vi "Vision Processing.vi"(4 "error in (no error)":errorcluster, 5 "Camera Type":enum16{"206", "1011"}(ring), 6 "Camera Name":string="Camera") -> (0 "Target Info":T1(array[cluster]), 2 "Processed Image":T3(plugin-control))   [LabVIEW 2013]
uses:
  Robot Global Data.vi
  <vilib>/vision/NI_Vision_Development_Module.lvlib
panel:
  in  "View":bool
  in  "Area Size Limit":i32=444
  in  "Particle Count Limit":i32=8
  in  "Score Limits":T2={"Rect Coverage"=76.0, "Aspect Ratio"=70.0, "X Edge Strength"=40.0, "Y Edge Strength"=60.0}
  in  "Processing":enum32{"Color", "Intensity", "Intensity Open"}(tab)
  in  "Luminance":i32=255
  in  "Saturation":i32=255
  in  "Hue":i32(knob)=65 scale=0.0..255.0
  in  "Margins":cluster{"Hue":i32, "Sat":i32, "Lum":i32}={"Hue"=20, "Sat"=27, "Lum"=30} {"Sat" scale=0.0..40.0; "Lum" scale=0.0..40.0; "Hue" scale=0.0..40.0}
  in  "Range":cluster{"Lower value":sgl, "Upper value":sgl}={"Lower value"=150.0, "Upper value"=255.0} {"Lower value" scale=0.0..255.0; "Upper value" scale=0.0..255.0}
  in  "Range":cluster{"Lower value":sgl, "Upper value":sgl}={"Lower value"=150.0, "Upper value"=255.0} {"Lower value" scale=0.0..255.0; "Upper value" scale=0.0..255.0}
  in  "View":bool
  out "Original Image":T3(plugin-control)
  # "Instructions:\nProcessing the reflective tape that is illuminated by a ring light can be based\non color or light intensity.\nParticles within the image are scored by rectangle coverage, aspect ratio, and\nfor being hollow with a bold edge. A particle is considered a target if all scores\nare above the score limits. Particles can be annotated -- surrounded by\na rectangle and scores drawn to the left .\nTo control the number of particles being scored, use the count limit and the size\nlimit."
  # "To debug, Enable using the View button.\nFor color processing, you can click in the image to select the color for processing."
  # "Enable by clicking the View button.\nGreen scores are above the limit, orange are below. Inner/outer rect\nindicates all passed."
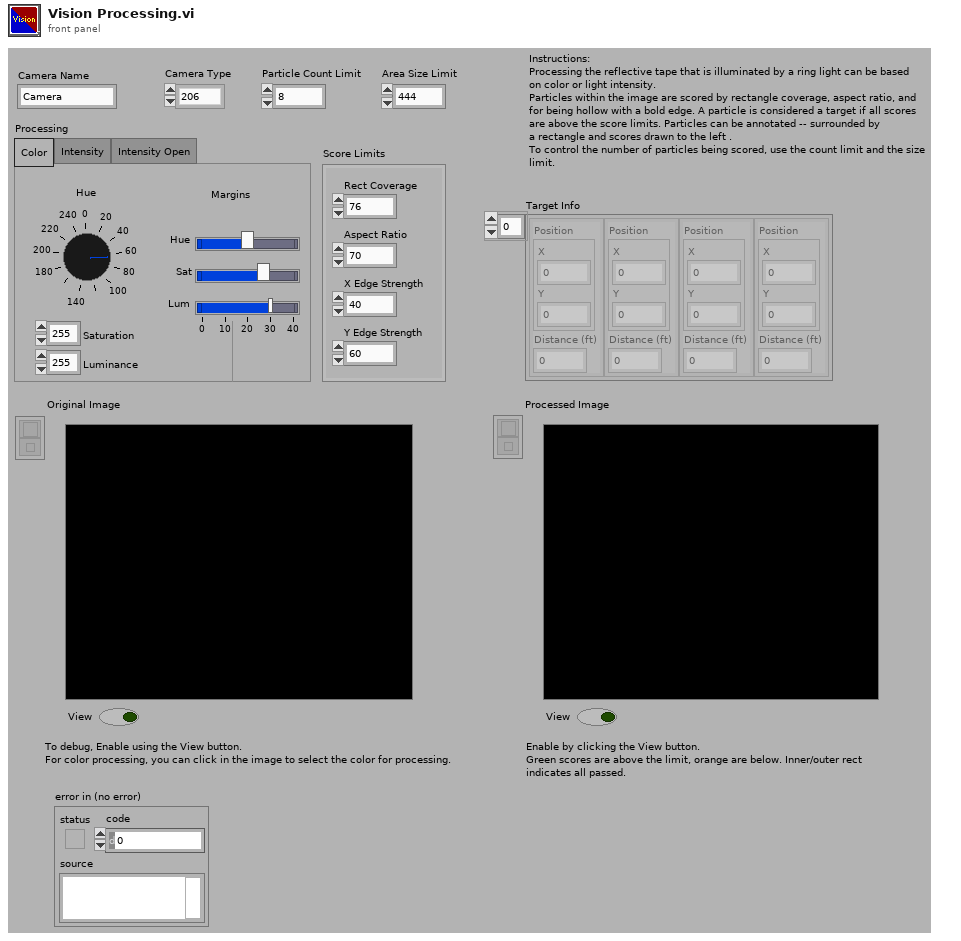
[diagram p1: front panel]
types:
  T1 = cluster{"Position":cluster{"X":dbl, "Y":dbl}, "Distance (ft)":dbl}[]
  T2 = cluster{"Rect Coverage":dbl, "Aspect Ratio":dbl, "X Edge Strength":dbl, "Y Edge Strength":dbl}
  T3 = typedef "IMAQ Image.ctl" = refnum<image>
  T4 = typedef "Image Type" = u32
  T5 = typedef "WPI_CameraDevRef.ctl" = cluster{"Camera Address":string, "CameraStatus":errorcluster, "Acquire Image Notifier":refnum<notifier>}
  T6 = enum32{"AutoM", "Close", "Dilate", "Erode", "Gradient", "Gradient out", "Gradient in", "Hit miss", "Open", "PClose", "POpen", "Thick", "Thin"}
  T7 = typedef "WPI_CameraImageSize.ctl" = enum16{"640x480", "320x240", "160x120"}
  T8 = cluster{cluster{"Left":dbl, "Top":dbl, "Right":dbl, "Bottom":dbl}, dbl[]}[]
  T9 = cluster{"Left":dbl, "Top":dbl, "Right":dbl, "Bottom":dbl}
  T10 = cluster{"Target Center (-1 to 1)":cluster{"X":dbl, "Y":dbl}, "Distance (ft)":dbl}
  T11 = cluster{"Target Center (-1 to 1)":cluster{"X":dbl, "Y":dbl}, "Distance (ft)":dbl}[]
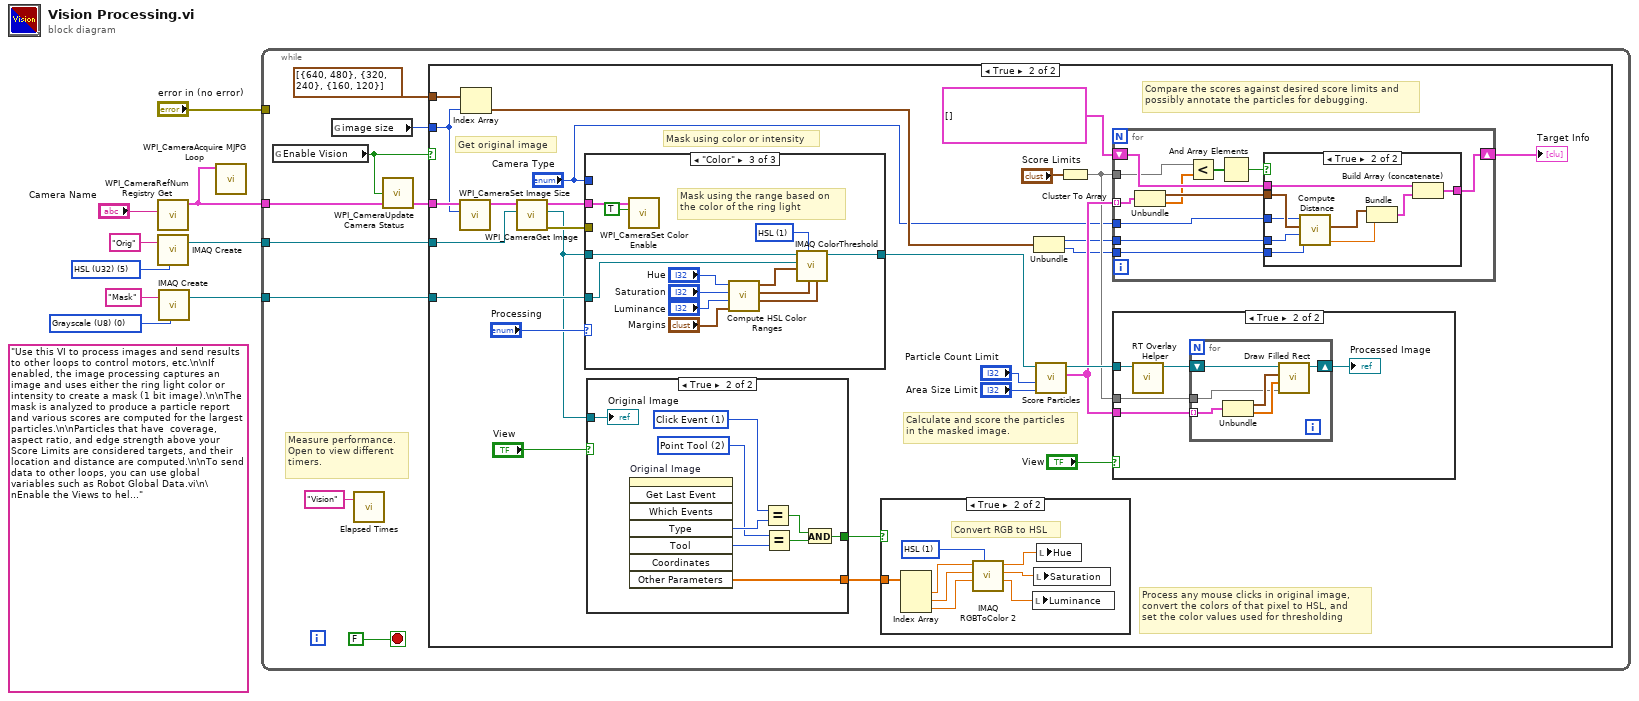
[diagram p0: block diagram]
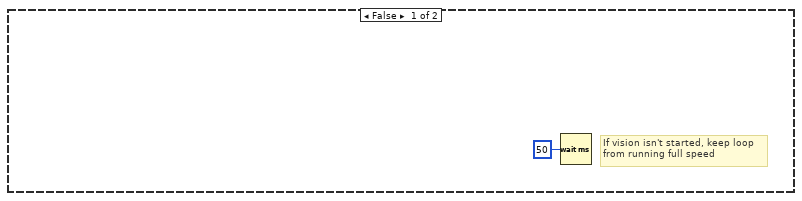
[diagram p2: hidden frame]
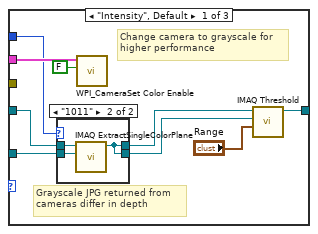
[diagram p4: hidden frame]
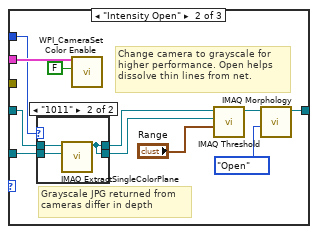
[diagram p6: hidden frame]
diagram:
  w3 = T4 0 items=["Grayscale (U8)", "Grayscale (I16)", "Grayscale (SGL)", "Complex (CSG)", "RGB (U32)", "HSL (U32)", "RGB (U64)", "Grayscale (U16)"] ("Image Type")
  (unwired) "Use this VI to process images and send results to other loops to control motors, etc.\n\nIf enabled, the image processing captures an image and uses either the ring light color or intensity to create a mask (1 bit image).\n\nThe mask is analyzed to produce a particle report and various scores are computed for the largest particles.\n\nParticles that have  coverage, aspect ratio, and edge strength above your Score Limits are considered targets, and their location and distance are computed.\n\nTo send data to other loops, you can use global variables such as Robot Global Data.vi\n\nEnable the Views to help debug color settings. Disable the View to speed up processing."
  w8 = T4 5 items=["Grayscale (U8)", "Grayscale (I16)", "Grayscale (SGL)", "Complex (CSG)", "RGB (U32)", "HSL (U32)", "RGB (U64)", "Grayscale (U16)"] ("Image Type")
  n1 = call <vilib>:"WPI_CameraRefNum Registry Get.vi"("refnum name"="Camera Name") -> ("CameraDevRef"=w5:T5)  [unwired: 9 in, 1 out]
  n2 = call "IMAQ Create"("Image Name"="Orig", "Image Type"=w8) -> ("New Image"=w7:T3)  [unwired: 2 in, 2 out]
  n3 = call "IMAQ Create"("Image Name"="Mask", "Image Type"=w3) -> ("New Image"=w1:T3)  [unwired: 2 in, 2 out]
  n4 = call <vilib>:"WPI_CameraAcquire MJPG Loop.vi"("CameraDevRef"=w5) -> ()  [unwired: 11 in]
  n5 = while {
    tunnel: w7 -> [w17]
    tunnel: w5 -> [w16]
    tunnel: "error in (no error)" -> [_]
    tunnel: w1 -> [w11]
    stop <- FALSE stop-if-true
    # "Measure performance.\nOpen to view different\ntimers."
    n6 = global read "Robot Global Data.vi" "Enable Vision"() -> (w14:bool)
    n7 = global read "Robot Global Data.vi" "image size"() -> (w12:T7)
    n8 = call "Elapsed Times.vi"("Call Name"="Vision") -> ()  [unwired: 2 in, 1 out]
    n9 = call <vilib>:"WPI_CameraUpdate Camera Status.vi"("CameraDevRef In"=w16, "Enable Vision"=w14) -> ("CameraDevRef Out"=w15:T5)  [unwired: 3 in]
    n10 = case shown="True" w14 {
      tunnel: w17 -> [_ w37]
      tunnel: w15 -> [_ w33]
      tunnel: w12 -> [_ w28]
      tunnel: w11 -> [_ w23]
      tunnel: cluster{i32, i32}[] [{640, 480}, {320, 240}, {160, 120}] -> [_ w27]
      frame False {
        # "If vision isn't started, keep loop\nfrom running full speed"
        n11 = Wait (ms)(milliseconds to wait=u32 50) -> ()  [unwired: 1 out]
      }
      frame True {
        # "Compare the scores against desired score limits and\npossibly annotate the particles for debugging."
        # "Process any mouse clicks in original image,\nconvert the colors of that pixel to HSL, and\nset the color values used for thresholding"
        # "Calculate and score the particles\nin the masked image."
        # "Mask using color or intensity"
        # "Get original image"
        n12 = call <vilib>:"WPI_CameraSet Image Size.vi"("Image Size"=w28, "CameraDevRef"=w33) -> ("CameraDevRef Out"=w34:T5)  [unwired: 8 in, 1 out]
        n13 = Index Array(array=w27, index=w28) -> (element=w24:cluster{i32, i32})
        n14 = call <vilib>:"WPI_CameraGet Image.vi"("Image"=w37, "CameraDevRef"=w34) -> ("error out"=w35:errorcluster, "Image Out"=w22:T3, "CameraDevRef Out"=w36:T5)  [unwired: 7 in]
        n15 = case shown="\"Color\"" "Processing" {
          tunnel: w22 -> [w59 w71 w97]
          tunnel: [w62 w76 w96] -> w31
          tunnel: w36 -> [w60 w74 w87]
          tunnel: w35 -> [_ _ _]
          tunnel: w23 -> [w58 w72 w85]
          tunnel: "Camera Type" -> [w57 w73 _]
          frame "Intensity", Default {
            # "Grayscale JPG returned from\ncameras differ in depth"
            # "Change camera to grayscale for\nhigher performance"
            n16 = case shown="\"1011\"" w57 {
              tunnel: w59 -> [w65 w68]
              tunnel: w58 -> [w64 w67]
              tunnel: [w65 w66] -> w56
              tunnel: [w64 w66] -> w55
              frame "206", Default {
              }
              frame "1011" {
                n17 = call "IMAQ ExtractSingleColorPlane"("Image Dst"=w67, "Image Src"=w68) -> ("Image Dst Out"=w66:T3)  [unwired: 8 in, 1 out]
              }
            }
            n18 = call <vilib>:"WPI_CameraSet Color Enable.vi"("Color Enabled"=FALSE, "CameraDevRef"=w60) -> ()  [unwired: 8 in, 2 out]
            n19 = call "IMAQ Threshold"("Range"="Range", "Image Dst"=w55, "Image Src"=w56) -> ("Image Dst Out"=w62:T3)  [unwired: 3 in, 5 out]
          }
          frame "Intensity Open" {
            # "Grayscale JPG returned from\ncameras differ in depth"
            # "Change camera to grayscale for\nhigher performance. Open helps\ndissolve thin lines from net."
            n20 = case shown="\"1011\"" w73 {
              tunnel: w71 -> [w81 w84]
              tunnel: w72 -> [w80 w83]
              tunnel: [w81 w82] -> w70
              tunnel: [w80 w82] -> w69
              frame "206", Default {
              }
              frame "1011" {
                n21 = call "IMAQ ExtractSingleColorPlane"("Image Dst"=w83, "Image Src"=w84) -> ("Image Dst Out"=w82:T3)  [unwired: 8 in, 1 out]
              }
            }
            n22 = call <vilib>:"WPI_CameraSet Color Enable.vi"("Color Enabled"=FALSE, "CameraDevRef"=w74) -> ()  [unwired: 8 in, 2 out]
            n23 = call "IMAQ Threshold"("Range"="Range", "Image Dst"=w69, "Image Src"=w70) -> ("Image Dst Out"=w77:T3)  [unwired: 3 in, 5 out]
            n24 = call "IMAQ Morphology"("Operation"=T6."Open", "Image Src"=w77) -> ("Image Dst Out"=w76:T3)  [unwired: 8 in, 1 out]
          }
          frame "Color" {
            w95 = u16 1 items=["RGB", "HSL", "HSV", "HSI"] ("Color Mode")
            # "Mask using the range based on\nthe color of the ring light"
            n25 = call <vilib>:"WPI_CameraSet Color Enable.vi"("Color Enabled"=TRUE, "CameraDevRef"=w87) -> ()  [unwired: 8 in, 2 out]
            n26 = call "Compute HSL Color Ranges.vi"("Margins"="Margins", "Luminance"="Luminance", "Saturation"="Saturation", "Hue"="Hue") -> ("Lum Range"=w92:cluster{i32, i32}, "Sat Range"=w93:cluster{i32, i32}, "Hue Range"=w94:cluster{i32, i32})  [unwired: 5 in]
            n27 = call "IMAQ ColorThreshold"("Blue or Luma or Val or Inten Range"=w92, "Green or Sat Range"=w93, "Color Mode"=w95, "Red or Hue Range"=w94, "Image Dst"=w85, "Image Src"=w97) -> ("Image Dst Out"=w96:T3)  [unwired: 4 in, 1 out]
          }
        }
        n28 = case shown="True" "View" {
          tunnel: w22 -> [_ w117]
          tunnel: [_ w112] -> w30
          tunnel: [_ w109] -> w29
          frame False {
          }
          frame True {
            w110 = 2 items=["None", "Selection Tool", "Point Tool", "Line Tool", "Rectangle Tool", "Oval Tool", "Polygon Tool", "ClosedFreehandTool", "Annulus Tool", "Rotated Rectangle Tool", "Zoom Tool", "Pan Tool", "Polyline Tool", "Freehand Tool"] ("Tool")
            w111 = 1 items=["No Event"=0, "Click Event"=1, "Draw Event"=2, "Size Event"=4, "Scroll Event"=5, "Double Click Event"=8] ("Type")
            n29 = invoke on="Original Image" class="ImageControl" method="Get Last Event"() -> ("Type"=w113:i32, "Tool"=w116:i32, "Other Parameters"=w109:sgl[])  [unwired: 8 in, 5 out]
            n30 = Equal?(x=w111, y=w113) -> (x = y?=w114:bool)
            n31 = Equal?(x=w110, y=w116) -> (x = y?=w115:bool)
            n32 = And(x=w114, y=w115) -> (x .and. y?=w112:bool)
            "Original Image" <- w117
          }
        }
        n33 = case shown="True" w30 {
          tunnel: w29 -> [_ w54]
          frame False {
          }
          frame True {
            w53 = u16 1 items=["RGB", "HSL", "HSV", "HSI", "CIE L*a*b*", "CIE XYZ"] ("Color Mode")
            # "Convert RGB to HSL"
            n34 = Index Array(array=w54) -> (element #1=w52:sgl, element #2=w50:sgl, element #3=w48:sgl)  [unwired: 3 in]
            n35 = call "IMAQ RGBToColor 2"("Color Mode"=w53, "Blue value"=w48, "Green value"=w50, "Red value"=w52) -> ("Blue or Luma or Val or Inten or Z or b*value"=w47:dbl, "Green or Sat or Y or a* value"=w49:dbl, "Red or Hue or X or L* value"=w51:dbl)  [unwired: 4 in, 1 out]
            n36 = local write "Luminance"(w47) -> ()
            n37 = local write "Saturation"(w49) -> ()
            n38 = local write "Hue"(w51) -> ()
          }
        }
        n39 = Unbundle(w24) -> (w26:i32, w25:i32)
        n40 = call "Score Particles.vi"("Area Size Limit"="Area Size Limit", "Particle Count Limit"="Particle Count Limit", "Image Refnum in"=w31) -> ("Scored Particle Info"=w42:T8, "Image Refnum out"=w45:T3)  [unwired: 7 in]
        n41 = Cluster To Array(cluster="Score Limits") -> (array=w40:dbl[])
        n42 = for {
          shift-right: [w127] -> w20
          shift-left: T1 [] -> [w128]
          tunnel: w26 -> [w126]
          tunnel: w42 -> [w124] mode=indexing
          tunnel: w40 -> [w119]
          tunnel: "Camera Type" -> [w123]
          tunnel: w25 -> [w118]
          n43 = Unbundle(w124) -> (w125:T9, w120:dbl[])
          n44 = Less?(x=w119, y=w120) -> (x < y?=w122:bool[])
          n45 = And Array Elements(Boolean array=w122) -> (logical AND=w121:bool)
          n46 = case shown="True" w121 {
            tunnel: w128 -> [w129 w138]
            tunnel: [w129 w137] -> w127
            tunnel: w125 -> [_ w133]
            tunnel: w126 -> [_ w135]
            tunnel: w123 -> [_ w132]
            tunnel: w118 -> [_ w131]
            frame False {
            }
            frame True {
              n47 = call "Compute Distance.vi"("Y Image Resolution"=w131, "X Image Resolution"=w135, "Bounding Box"=w133, "Camera Type"=w132) -> ("Target Center (-1 to 1)"=w130:cluster{"X":dbl, "Y":dbl}, "Distance (ft)"=w134:dbl)  [unwired: 6 in]
              n48 = Bundle("Target Center (-1 to 1)"=w130, "Distance (ft)"=w134) -> (w136:T10)  [unwired: 1 in]
              n49 = Build Array (concatenate)(w138, w136) -> (w137:T11)
            }
          }
        }
        "Target Info" <- w20
        n50 = case shown="True" "View" {
          tunnel: w45 -> [_ w99]
          tunnel: w42 -> [_ w101]
          tunnel: w40 -> [_ w100]
          frame False {
          }
          frame True {
            n51 = call "RT Overlay Helper.vi"("Refnum in"=w99) -> ("Refnum out"=w102:T3)  [unwired: 10 in]
            n52 = for {
              shift-right: [w107] -> w98
              shift-left: w102 -> [w108]
              tunnel: w101 -> [w104] mode=indexing
              tunnel: w100 -> [w103]
              n53 = Unbundle(w104) -> (w105:T9, w106:dbl[])
              n54 = call "Draw Filled Rect.vi"("Limits"=w103, "Scores"=w106, "Bounding Box"=w105, "image in"=w108) -> ("image out"=w107:T3)  [unwired: 7 in]
            }
            "Processed Image" <- w98
          }
        }
      }
    }
  }
